vi "MagnetControl.vi"(8 "error in (no error)":errorcluster, 11 "VISA resource name":refnum<visa-resource-name>="iPS") -> (0 "error out":errorcluster)   [LabVIEW 2021]
uses:
  controls/iPSreadCtrl.ctl
  controls/iPSsetCtrl.ctl
  <vilib>/Utility/file.llb/Write Delimited Spreadsheet (string).vi
panel:
  in  "FilePath":path
  in  "Every (s)":dbl=60.0
  in  "Save Log":bool
  out "Monitor":T1(graph)
  in  "Target Field, T":dbl min=-18.0 max=18.0 step=0.01
  in  "iPSSetCtrl":T2
  in  "Field Rate, T/min":dbl min=0.0 max=0.2 step=0.0001
  out "Magnet Readings":T3={"Signals"=["Output Field (T)", "Magnet Field (T)", "Switch Heater Temp (K)", "Field Rate (T/min)", "Magnet Temp (T)"], "Magnet Readings"=[0.0, -1.2307692307692308e-05, 291.0928, 0.1, 290.5584]}
  in  "iPSreadCtrl":T4=enum."Switch Heater Temp"
  in  "Set":bool
  in  "Refresh Time (ms)":i32=100
  in  "Quit":bool
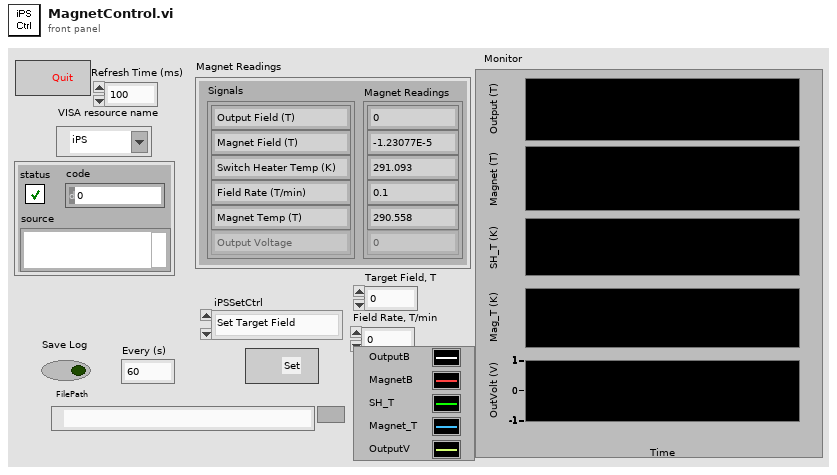
[diagram p1: front panel]
types:
  T1 = cluster{"number":dbl, "number":dbl, "number":dbl, "number":dbl, "number":dbl}
  T2 = typedef "iPSsetCtrl.ctl" = enum16{"Set Target Field", "Set Target Field Rate", "Switch Heater ON", "Switch Heater OFF", "Go to Field", "Go to Zero", "Hold"}
  T3 = cluster{"Signals":string[], "Magnet Readings":dbl[]}
  T4 = typedef "iPSreadCtrl.ctl" = enum16{"OutputField", "MagnetField", "Switch Heater Temp", "Field Rate", "Magnet Temp", "OutputVoltage"}
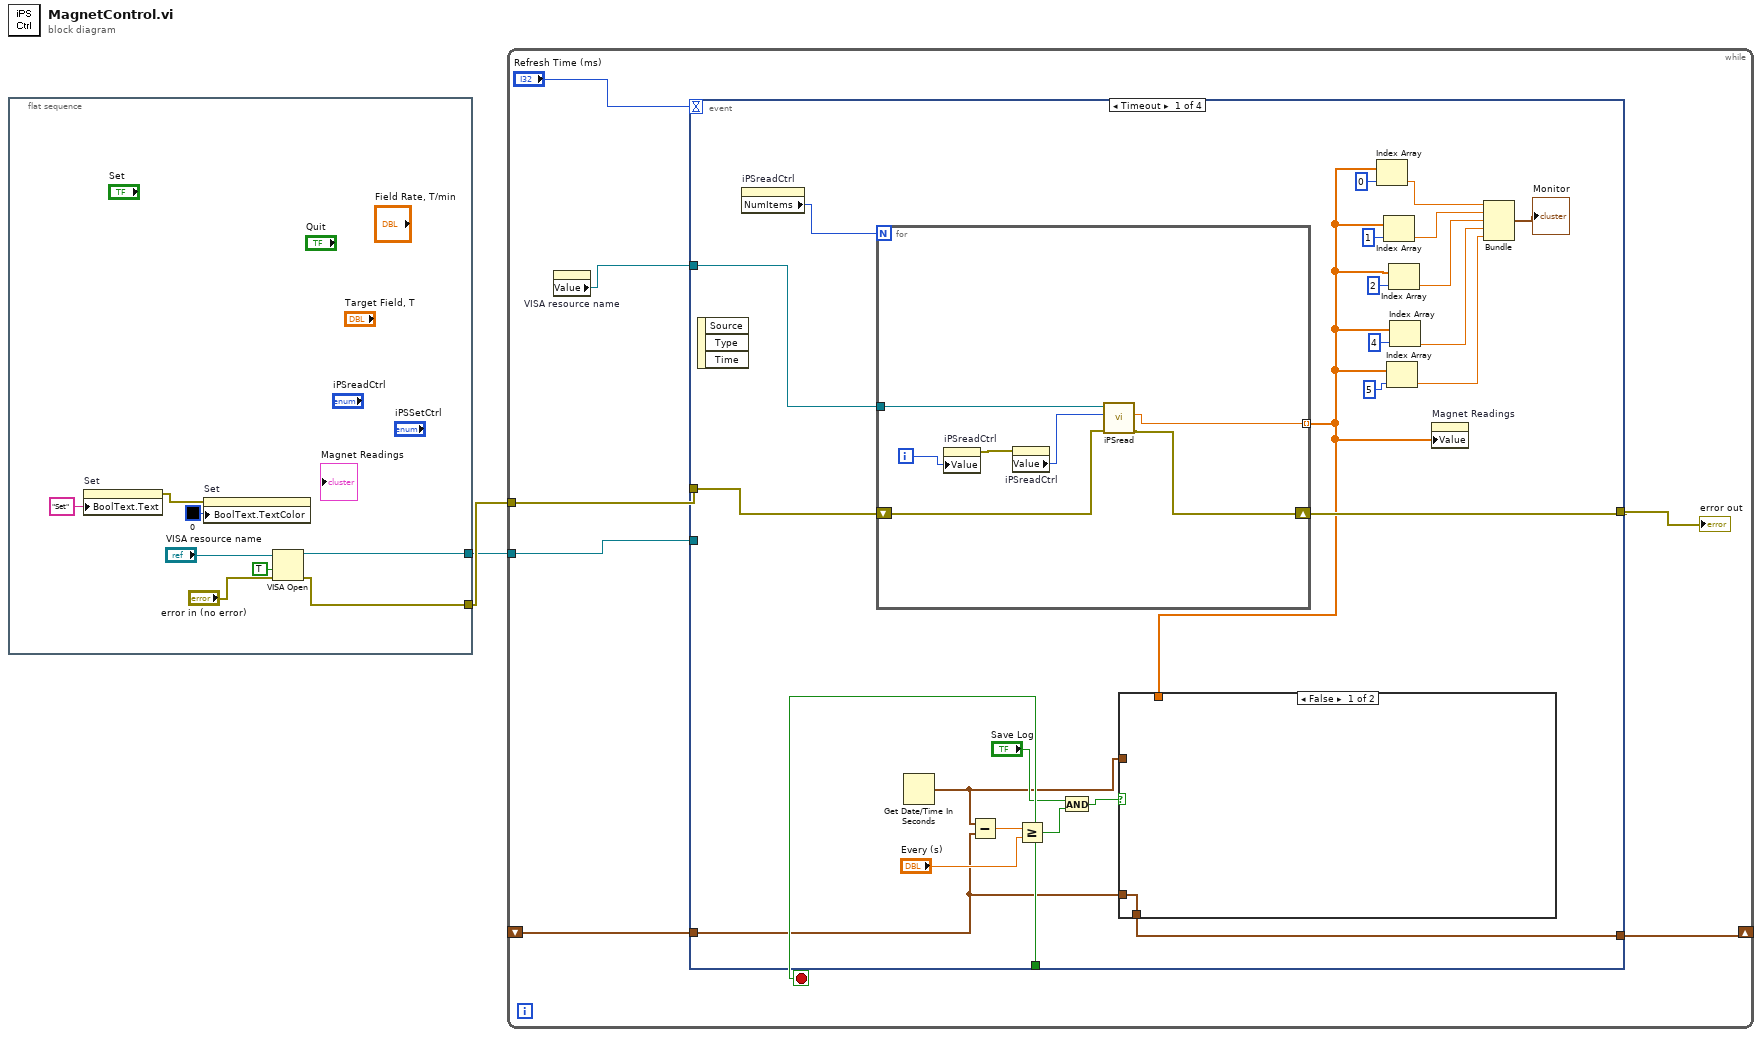
[diagram p0: block diagram]
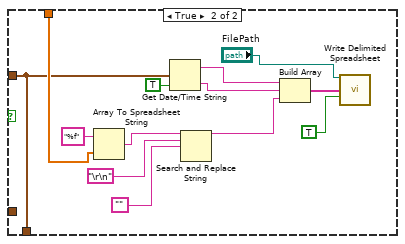
[diagram p2: hidden frame]
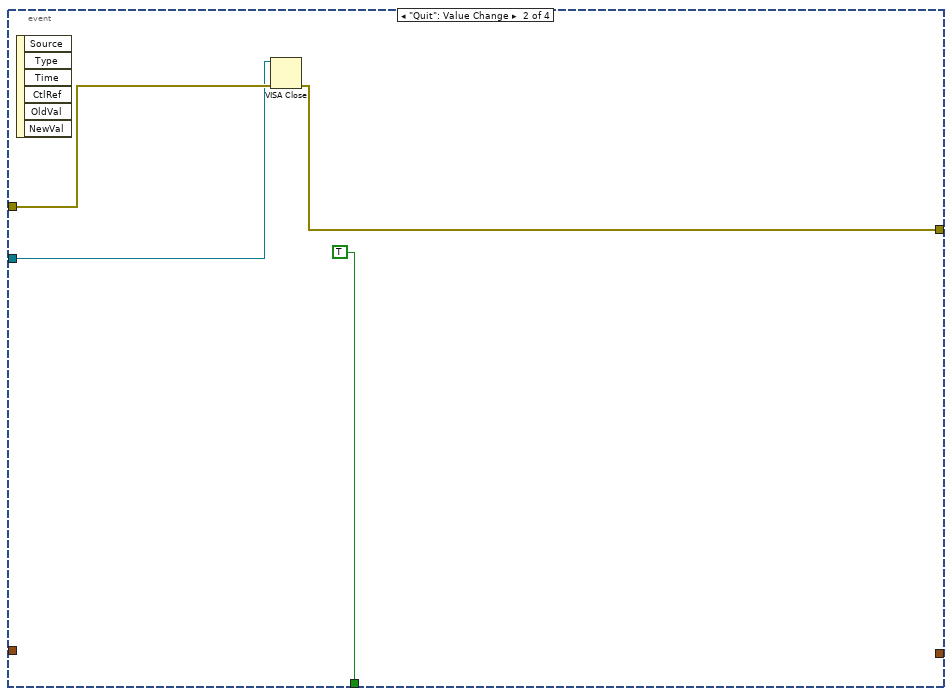
[diagram p3: hidden frame]
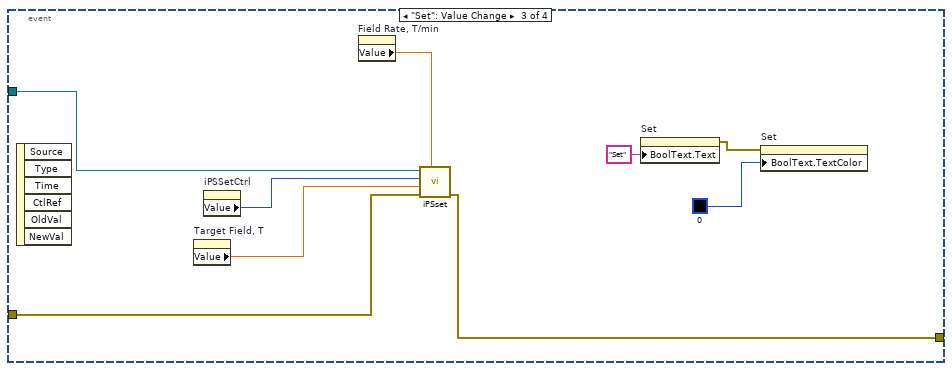
[diagram p4: hidden frame]
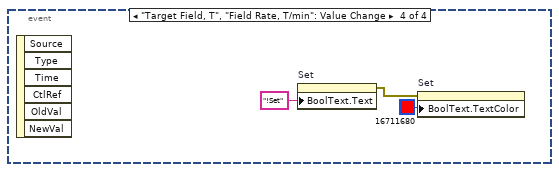
[diagram p5: hidden frame]
diagram:
  n1 = flat-sequence {
    tunnel: [w5] -> w2
    tunnel: [w3] -> w1
    frame #0 {
      n2 = property on="Set" class="Bool (strict)"("BoolText.Text"="Set" ("Boolean Text.Text")) -> (error out=w10:errorcluster)  [unwired: 2 in, 1 out]
      n3 = property on="Set" class="Bool (strict)"(error in=w10, "BoolText.TextColor"=u32 0 ("Boolean Text.Colors:BG Color")) -> ()  [unwired: 1 in, 2 out]
      n4 = VISA Open(duplicate session (F)=TRUE, error in (no error)="error in (no error)", VISA resource name="VISA resource name") -> (VISA resource name=w3:refnum<visa-resource-name>, error out=w5:errorcluster)  [unwired: 2 in]
    }
  }
  n5 = while {
    tunnel: w2 -> [w17]
    tunnel: w1 -> [w14]
    shift-right: [w12] -> _
    shift-left: _ -> [w11]
    stop <- w16 stop-if-true
    n6 = property on="VISA resource name" class="VISAName"() -> ("Value"=w13:refnum<visa-resource-name>)  [unwired: 2 in, 2 out]
    n7 = event shown="[0] Timeout" {
      selector: _ -> [_ _ _ _]
      dyn-events: _ -> [_ _ _ _]
      timeout: "Refresh Time (ms)" -> [_ _ _ _]
      tunnel: w17 -> [w42 w66 w70 _]
      tunnel: [w41 w65 w69 _] -> w15
      tunnel: [_ TRUE _ _] -> w16
      tunnel: w14 -> [_ w64 _ _]
      tunnel: w13 -> [w30 _ w68 _]
      tunnel: [w27 _ _ _] -> w12
      tunnel: w11 -> [w22 _ _ _]
      event Timeout {
        n8 = event-data() -> ()  [unwired: 1 in, 3 out]
        n9 = property on="iPSreadCtrl" class="Enum (strict)"() -> ("NumItems"=w40:u32)  [unwired: 2 in, 2 out]
        n10 = for {
          N: w40 -> [_]
          shift-right: [w62] -> w41
          shift-left: w42 -> [w63]
          tunnel: [w61] -> w21 mode=indexing
          tunnel: w30 -> [w57]
          i -> [w60]
          n11 = property on="iPSreadCtrl" class="Enum (strict)"("Value"=w60) -> (error out=w59:errorcluster)  [unwired: 2 in, 1 out]
          n12 = property on="iPSreadCtrl" class="Enum (strict)"(error in=w59) -> ("Value"=w58:T4)  [unwired: 1 in, 2 out]
          n13 = call "iPSread.vi"("error in (no error)"=w63, "iPSreadCtrl"=w58, "VISA resource name"=w57) -> ("error out"=w62:errorcluster, "number"=w61:dbl)  [unwired: 5 in, 2 out]
        }
        n14 = Get Date/Time In Seconds() -> (seconds since 1Jan1904=w26:timestamp)
        n15 = Subtract(x=w26, y=w22) -> (x-y=w24:dbl)
        n16 = Greater Or Equal?(x=w24, y="Every (s)") -> (x >= y?=w23:bool)
        n17 = And(x="Save Log", y=w23) -> (x .and. y?=w28:bool)
        n18 = case shown="False" w28 {
          tunnel: w26 -> [_ w51]
          tunnel: [w43 w51] -> w27
          tunnel: w22 -> [w43 _]
          tunnel: w21 -> [_ w56]
          frame False {
          }
          frame True {
            n19 = Array To Spreadsheet String(array=w56, 3:"%f" ("format string")) -> (spreadsheet string=w54:string)  [unwired: 1 in]
            n20 = Get Date/Time String(seconds (now)=w51, want seconds? (F)=TRUE ("UTC format")) -> (date string=w49:string, time string=w48:string)  [unwired: 1 in]
            n21 = Search and Replace String(input string=w54, search string="\r\n", replace string="" ("replace string (\"\")")) -> (result string=w47:string)  [unwired: 5 in, 3 out]
            n22 = Build Array(w49, w48, w47) -> (w46:string[])
            n23 = call-poly <vilib>:"Write Delimited Spreadsheet.vi"("file path (dialog if empty)"="FilePath", "1D data"=w46, "append to file? (new file:F)"=TRUE) -> ()  [unwired: 11 in, 2 out]
          }
        }
        n24 = Index Array(array=w21, index=0) -> (element=w36:dbl)
        n25 = Index Array(array=w21, index=1) -> (element=w34:dbl)
        n26 = Index Array(array=w21, index=5) -> (element=w19:dbl)
        n27 = Index Array(array=w21, index=2) -> (element=w31:dbl)
        n28 = Index Array(array=w21, index=4) -> (element=w33:dbl)
        n29 = property on="Magnet Readings" class="Arr (strict)"("Value"=w21) -> ()  [unwired: 2 in, 2 out]
        n30 = Bundle("number"=w36, "number"=w34, "number"=w31, "number"=w33, "number"=w19) -> (→"Monitor":T1)  [unwired: 1 in]
      }
      event "Quit": Value Change {
        n31 = event-data() -> ()  [unwired: 1 in, 6 out]
        n32 = VISA Close(VISA resource name=w64, error in (no error)=w66) -> (error out=w65:errorcluster)
      }
      event "Set": Value Change {
        n33 = event-data() -> ()  [unwired: 1 in, 6 out]
        n34 = property on="Target Field, T" class="DigNum (strict)"() -> ("Value"=w71:dbl)  [unwired: 2 in, 2 out]
        n35 = property on="iPSSetCtrl" class="Enum (strict)"() -> ("Value"=w72:T2)  [unwired: 2 in, 2 out]
        n36 = property on="Field Rate, T/min" class="DigNum (strict)"() -> ("Value"=w73:dbl)  [unwired: 2 in, 2 out]
        n37 = call "iPSset.vi"("Field Rate, T/min"=w73, "error in (no error)"=w70, "Target Field, T"=w71, "iPSSetCtrl"=w72, "VISA resource name"=w68) -> ("error out"=w69:errorcluster)  [unwired: 3 in, 3 out]
        n38 = property on="Set" class="Bool (strict)"("BoolText.Text"="Set" ("Boolean Text.Text")) -> (error out=w74:errorcluster)  [unwired: 2 in, 1 out]
        n39 = property on="Set" class="Bool (strict)"(error in=w74, "BoolText.TextColor"=u32 0 ("Boolean Text.Colors:BG Color")) -> ()  [unwired: 1 in, 2 out]
      }
      event "Target Field, T", "Field Rate, T/min": Value Change {
        n40 = event-data() -> ()  [unwired: 1 in, 6 out]
        n41 = property on="Set" class="Bool (strict)"("BoolText.Text"="!Set" ("Boolean Text.Text")) -> (error out=w78:errorcluster)  [unwired: 2 in, 1 out]
        n42 = property on="Set" class="Bool (strict)"(error in=w78, "BoolText.TextColor"=u32 16711680 ("Boolean Text.Colors:BG Color")) -> ()  [unwired: 1 in, 2 out]
      }
    }
    "error out" <- w15
  }
